vi "ErrorCaseString.vi"(5 "Error":string, 6 "selector string":string, 7 "No Error":string) -> (1 "Default":bool, 4 "case":string)   [LabVIEW 2014, in "CaseStructure.lvclass"]
uses:
  CaseStructure.lvclass
  Python/Parsing/ListTypesTD.ctl
  Python/Parsing/Python Functions.lvlib
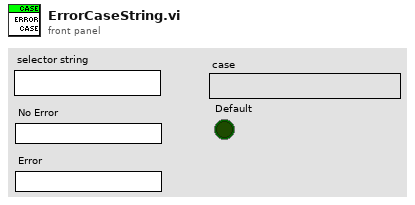
[diagram p1: front panel]
types:
  T1 = typedef "Python Functions.lvlib/ListTypesTD.ctl" = enum16{"list", "tuple", "parameter list", "output list", "return values"}
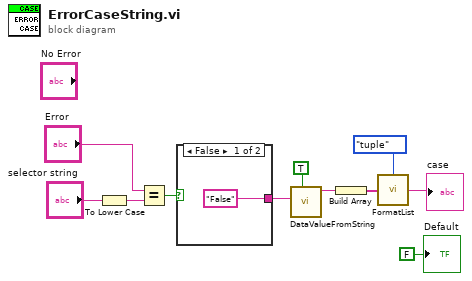
[diagram p0: block diagram]
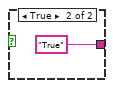
[diagram p2: hidden frame]
diagram:
  n1 = To Lower Case(string="selector string") -> (all lower case string=w3:string)
  n2 = Equal?(x="Error", y=w3) -> (x = y?=w1:bool)
  n3 = case shown="False" w1 {
    tunnel: ["False" "True"] -> w4
    frame False {
    }
    frame True {
    }
  }
  n4 = call "DataValueFromString.vi"("Type"=TRUE, "value"=w4) -> ("value"=w8:string)  [unwired: 7 in]
  n5 = Build Array(w8) -> (w7:string[])
  n6 = call "FormatList.vi"("values"=w7, "type"=ListTypesTD."tuple") -> ("python object"=→"case":string)
  "Default" <- FALSE ("Default")
